vi "LVDimInterface.application example client.vi"() -> ()   [LabVIEW 2015, in "LVDimInterface.lvlib"]
doc: "This is an example of a DIM client receiving service data via a message queue."
uses:
  LVDimInterface.lvlib
  <vilib>/Utility/miscctls.llb/LVDateTimeRec.ctl
  LVDimInterface.dim service type.ctl
  LVDimInterface.dic_info_service_queue.vi
panel:
  out "date time rec":T1
  out "error out":errorcluster
  out "callBackID":i32=1
  out "no link":bool
  out "serviceData":i32=1313819721
  out "serviceSize":i32=4
  in  "serviceName":string="testService"
  out "receivedCounter":i32=1
  in  "stop":bool
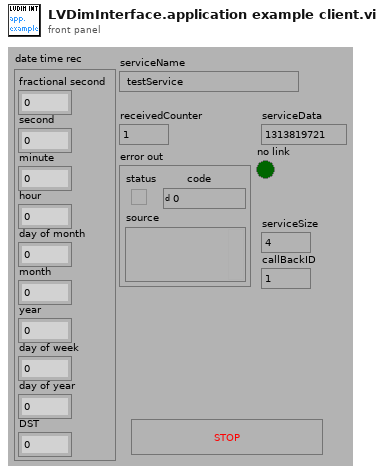
[diagram p1: front panel]
types:
  T1 = typedef "LVDateTimeRec.ctl" = cluster{"fractional second":dbl, "second":i32, "minute":i32, "hour":i32, "day of month":i32, "month":i32, "year":i32, "day of week":i32, "day of year":i32, "DST":i32}
  T2 = typedef "LVDimInterface.lvlib/LVDimInterface.dim service type.ctl" = u16
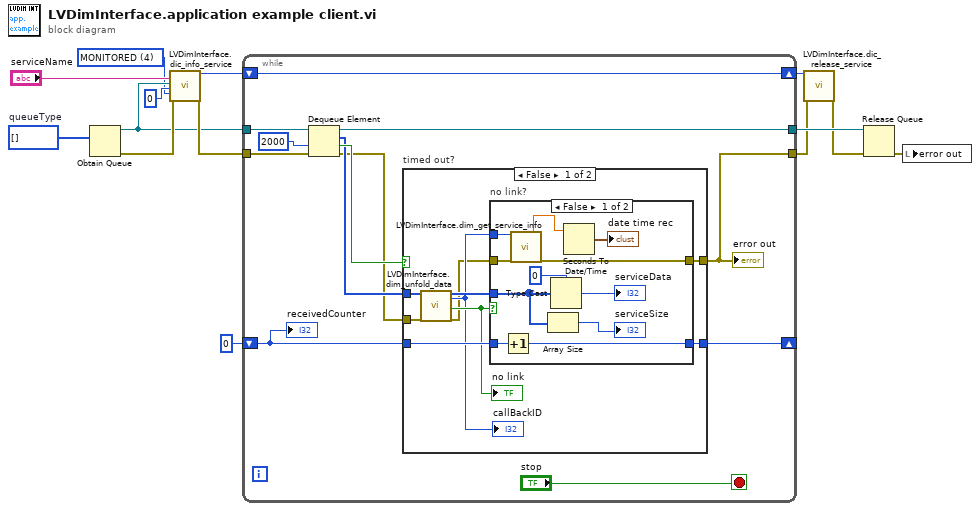
[diagram p0: block diagram]
diagram:
  w2 = T2 4 items=["ONCE_ONLY"=1, "TIMED"=2, "MONITORED"=4] ("serviceType")
  w5 = i8[] []  # queueType
  n1 = Obtain Queue(element data type=w5) -> (queue out=w4:refnum<queue>, error out=w11:errorcluster)  [unwired: 4 in, 1 out]
  n2 = call-poly "LVDimInterface.dic_info_service.vi"("serviceName"="serviceName", "queueRef"=w4, "timeout [s]"=0, "serviceType"=w2, "error in (no error)"=w11) -> ("callBackID"=w14:i32, "error out"=w10:errorcluster)  [unwired: 13 in]
  n3 = while {
    tunnel: w4 -> [w26]
    tunnel: [w24] -> w13
    shift-right: [w20] -> _
    shift-left: 0 -> [w21]
    tunnel: w10 -> [w19]
    tunnel: [w15] -> w8
    shift-right: [w17] -> w9
    shift-left: w14 -> [w17]
    stop <- "stop" stop-if-true
    n4 = Dequeue Element(queue=w26, timeout in ms (-1)=2000, error in (no error)=w19) -> (queue out=w24:refnum<queue>, element=w18:i8[], timed out?=w23:bool, error out=w16:errorcluster)
    n5 = case "timed out?" shown="False" w23 {
      tunnel: [w34 w50] -> w20
      tunnel: w21 -> [w35 w50]
      tunnel: w18 -> [w32 _]
      tunnel: w16 -> [w29 w49]
      tunnel: [w27 w49] -> w15
      frame False {
        n6 = call "LVDimInterface.dim_unfold_data.vi"("rawData"=w32, "error in (no error)"=w29) -> ("data"=w33:i8[], "callBackID"=w30:i32, "no link"=w31:bool, "error out"=w28:errorcluster)  [unwired: 14 in]
        "no link" <- w31
        "callBackID" <- w30
        n7 = case "no link?" shown="False" w31 {
          tunnel: w35 -> [w46 w48]
          tunnel: [w45 w48] -> w34
          tunnel: w33 -> [w42 _]
          tunnel: w30 -> [w40 _]
          tunnel: w28 -> [w37 w47]
          tunnel: [w36 w47] -> w27
          frame False {
            n8 = Increment(x=w46) -> (x+1=w45:i32)
            n9 = call "LVDimInterface.dim_get_service_info.vi"("callBackID"=w40, "error in (no error)"=w37) -> ("timeStamp"=w38:dbl, "error out"=w36:errorcluster)  [unwired: 8 in, 8 out]
            n10 = Array Size(array=w42) -> (size(s)=→"serviceSize":i32)
            n11 = Type Cast(type=0, x=w42) -> (*(type *) &x=→"serviceData":i32)
            n12 = Seconds To Date/Time(time stamp (now)=w38) -> (date time rec=→"date time rec":T1)  [unwired: 1 in]
          }
          frame True {
          }
        }
      }
      frame True {
      }
    }
    "error out" <- w15
    "receivedCounter" <- w21
  }
  n13 = call "LVDimInterface.dic_release_service.vi"("callBackID"=w9, "error in (no error)"=w8) -> ("error out"=w7:errorcluster)  [unwired: 17 in]
  n14 = Release Queue(queue=w13, error in (no error)=w7) -> (error out=w1:errorcluster)  [unwired: 1 in, 2 out]
  n15 = local write "error out"(w1) -> ()
